vi "Table, Import from Excel Clipboard.vi"(8 "error in":errorcluster, 10 "Excel Clipboard to Import":string="TRS13058\tPower Test\t\t\t\t\nTRS13059\tAdapter Source Regulator Test \t\t\t\t\nTRS13060\t+3.3\t3.135\t3.465\tVDC\tGELE\nTRS13061\t+3.3_CONT\t3.135\t3.465\tVDC\tGELE\nTRS13062\tIVAD, ADAPTER Power Supply Current\t30\t40\tmA\tGELE\nTRS13063\tExternal Battery Source Regulator Test \t\t\t\t\nTRS13064\t+3.3\t3.135\t3.465\tVDC\tGELE\nTRS13065\t+3.3_CONT\t3.135\t3.465\tVDC\tGELE\nTRS13066\tIEXTBATT, EXT_BAT Power Supply Current\t35\t45\tmA\tGELE\nTRS13067\tInternal Battery Source Regulator Test \t\t\t\t\nTRS13068\t+3.3\t3.135\t3.465\tVDC\tGELE\nTRS13069\t+3.3_CONT\t3.135\t3.465\tVDC\tGELE\nTRS13070\tIINTBATT, INT_BAT Power Supply Current\t40\t50\tmA\tGELE\nTRS13071\t3.3V_ANALOG\t3.135\t3.465\tVDC\tGELE\nTRS13259\tReset Test\t\t\t\t\nTRS13260\tBC_RST with MR_BC_RST High\t1\t\tTTL\tEQ\nTRS13261\tBC_RST with MR_BC_RST Low\t0\t\tTTL\tEQ\nTRS13262\tMC_RST with MR_MC_RST High\t1\t\tTTL\tEQ\nTRS13263\tMC_RST with MR_MC_RST Low\t0\t\tTTL\tEQ\nTRS13072\tPower Switching\t\t\t\t\nTRS13073\tAdapter Source \t\t\t\t\nTRS13074\tVSYS\t17.1\t18.9\tVDC\tGELE\nTRS13075\tIVAD, ADAPTER Power Supply Current\t30\t40\tmA\tGELE\nTRS13076\tIEXTBATT, EXT_BAT Power Supply Current\t0\t10\tmA\tGELE\nTRS13077\tIINTBATT, INT_BAT Power Supply Current\t0\t10\tmA\tGELE\nTRS13078\tExternal Battery Source 16.8 V\t\t\t\t\nTRS13079\tVSYS\t15.96\t17.64\tVDC\tGELE\nTRS13080\tIVAD, ADAPTER Power Supply Current\t0\t10\tmA\tGELE\nTRS13081\tIEXTBATT, EXT_BAT Power Supply Current\t35\t45\tmA\tGELE\nTRS13082\tIINTBATT, INT_BAT Power Supply Current\t0\t10\tmA\tGELE\nTRS13083\tInternal Battery Source 16 V\t\t\t\t\nTRS13084\tVSYS\t15.2\t16.8\tVDC\tGELE\nTRS13085\tIVAD, ADAPTER Power Supply Current\t0\t10\tmA\tGELE\nTRS13086\tIEXTBATT, EXT_BAT Power Supply Current\t0\t10\tmA\tGELE\nTRS13087\tIINTBATT, INT_BAT Power Supply Current\t40\t50\tmA\tGELE\nTRS13109\tExternal Battery Source 16.8 V (repeat 3.3.2)\t\t\t\t\nTRS13110\tVSYS\t15.96\t17.64\tVDC\tGELE\nTRS13111\tIVAD, ADAPTER Power Supply Current\t0\t10\tmA\tGELE\nTRS13112\tIEXTBATT, EXT_BAT Power Supply Current\t25\t45\tmA\tGELE\nTRS13113\tIINTBATT, INT_BAT Power Supply Current\t0\t10\tmA\tGELE\nTRS13088\tExternal Battery Source 14.8 V\t\t\t\t\nTRS13089\tVSYS\t14.06\t15.54\tVDC\tGELE\nTRS13090\tIVAD, ADAPTER Power Supply Current\t0\t10\tmA\tGELE\nTRS13091\tIEXTBATT, EXT_BAT Power Supply Current\t40\t50\tmA\tGELE\nTRS13092\tIINTBATT, INT_BAT Power Supply Current\t0\t10\tmA\tGELE\nTRS13093\tExternal Battery Source 12.8 V\t\t\t\t\nTRS13094\tVSYS\t12.16\t13.44\tVDC\tGELE\nTRS13095\tIVAD, ADAPTER Power Supply Current\t0\t10\tmA\tGELE\nTRS13096\tIEXTBATT, EXT_BAT Power Supply Current\t45\t60\tmA\tGELE\nTRS13097\tIINTBATT, INT_BAT Power Supply Current\t0\t10\tmA\tGELE\nTRS13098\tInternal Battery Source 14 V\t\t\t\t\nTRS13099\tVSYS\t13.3\t14.7\tVDC\tGELE\nTRS13100\tIVAD, ADAPTER Power Supply Current\t0\t10\tmA\tGELE\nTRS13101\tIEXTBATT, EXT_BAT Power Supply Current\t0\t10\tmA\tGELE\nTRS13102\tIINTBATT, INT_BAT Power Supply Current\t45\t60\tmA\tGELE\nTRS13103\tInternal Battery Source 12 V\t\t\t\t\nTRS13104\tVSYS\t11.4\t12.6\tVDC\tGELE\nTRS13105\tIVAD, ADAPTER Power Supply Current\t0\t10\tmA\tGELE\nTRS13106\tIEXTBATT, EXT_BAT Power Supply Current\t0\t10\tmA\tGELE\nTRS13107\tIINTBATT, INT_BAT Power Supply Current\t50\t65\tmA\tGELE\nTRS13267\tDormant Mode Operation\t\t\t\t\nTRS13268\tInternal Battery Source 16 V\t\t\t\t\nTRS13269\tVSYS\t15.2\t16.8\tVDC\tGELE\nTRS13270\tIVAD, ADAPTER Power Supply Current\t0\t10\tmA\tGELE\nTRS13271\tIEXTBATT, EXT_BAT Power Supply Current\t0\t10\tmA\tGELE\nTRS13272\tIINTBATT, INT_BAT Power Supply Current\t40\t50\tmA\tGELE\nTRS13273\tDormant Mode\t\t\t\t\nTRS13274\tVSYS\t-0.5\t0.5\tVDC\tGELE\nTRS13275\t+3.3_CONT\t3.135\t3.465\tVDC\tGELE\nTRS13469\tExternal Power Detect\t\t\t\t\nTRS13470\tAdapter Detect\t1\t\tTTL\tEQ\nTRS13471\tEXT_BAT Detect\t1\t\tTTL\tEQ\nTRS13472\tINT_BAT Detect\t0\t\tTTL\tEQ\nTRS13108\tBooster Check\t\t\t\t\nTRS13114\tAdapter Source \t\t\t\t\nTRS13115\tVMOTOR with 0.25A Load\t17.1\t18.9\tVDC\tGELE\nTRS13264\tVMOTOR_DRIVER with 0.25A Load\t12.04\t12.54\tVDC\tGELE\nTRS13116\tVMOTOR with 0.5A Load\t17.1\t18.9\tVDC\tGELE\nTRS13265\tVMOTOR_DRIVER with 0.5A Load\t12.04\t12.54\tVDC\tGELE\nTRS13117\tVMOTOR with 1.0A Load\t17.1\t18.9\tVDC\tGELE\nTRS13266\tVMOTOR_DRIVER with 1.0A Load\t12.04\t12.54\tVDC\tGELE\nTRS13118\tExternal Battery Source 16.8 V\t\t\t\t\nTRS13119\tVMOTOR with 0.25A Load\t17.64\t18.36\tVDC\tGELE\nTRS13120\tVMOTOR with 0.5A Load\t17.64\t18.36\tVDC\tGELE\nTRS13121\tVMOTOR with 1.0A Load\t17.64\t18.36\tVDC\tGELE\nTRS13122\tInternal Battery Source 16 V\t\t\t\t\nTRS13123\tVMOTOR with 0.25A Load\t17.64\t18.36\tVDC\tGELE\nTRS13124\tVMOTOR with 0.5A Load\t17.64\t18.36\tVDC\tGELE\nTRS13125\tVMOTOR with 1.0A Load\t17.64\t18.36\tVDC\tGELE\nTRS13126\tExternal Battery Source 16.8 V\t\t\t\t\nTRS13127\tVMOTOR with 0.25A Load\t17.64\t18.36\tVDC\tGELE\nTRS13128\tVMOTOR with 0.5A Load\t17.64\t18.36\tVDC\tGELE\nTRS13129\tVMOTOR with 1.0A Load\t17.64\t18.36\tVDC\tGELE\nTRS13130\tExternal Battery Source 14.8 V\t\t\t\t\nTRS13131\tVMOTOR with 0.25A Load\t17.64\t18.36\tVDC\tGELE\nTRS13132\tVMOTOR with 0.5A Load\t17.64\t18.36\tVDC\tGELE\nTRS13133\tVMOTOR with 1.0A Load\t17.64\t18.36\tVDC\tGELE\nTRS13134\tExternal Battery Source 12.8 V\t\t\t\t\nTRS13135\tVMOTOR with 0.25A Load\t17.64\t18.36\tVDC\tGELE\nTRS13136\tVMOTOR with 0.5A Load\t17.64\t18.36\tVDC\tGELE\nTRS13137\tVMOTOR with 1.0A Load\t17.64\t18.36\tVDC\tGELE\nTRS13138\tInternal Battery Source 14 V\t\t\t\t\nTRS13139\tVMOTOR with 0.25A Load\t17.64\t18.36\tVDC\tGELE\nTRS13140\tVMOTOR with 0.5A Load\t17.64\t18.36\tVDC\tGELE\nTRS13141\tVMOTOR with 1.0A Load\t17.64\t18.36\tVDC\tGELE\nTRS13142\tInternal Battery Source 12 V\t\t\t\t\nTRS13143\tVMOTOR with 0.25A Load\t17.64\t18.36\tVDC\tGELE\nTRS13144\tVMOTOR with 0.5A Load\t17.64\t18.36\tVDC\tGELE\nTRS13145\tVMOTOR with 1.0A Load\t17.64\t18.36\tVDC\tGELE\nTRS13146\tAdapter Source (repeat step 3.6.1?)\t\t\t\t\nTRS13147\tVMOTOR with 0.25A Load\t17.64\t18.36\tVDC\tGELE\nTRS13148\tVMOTOR with 0.5A Load\t17.64\t18.36\tVDC\tGELE\nTRS13149\tVMOTOR with 1.0A Load\t17.64\t18.36\tVDC\tGELE\nTRS13633\tMotor Driver Test\t\t\t\t\nTRS13634\tStator A Phase U and Phase V\t\t\t\t\nTRS13635\tPhase U to V\t17.64\t18.36\tVDC\tGELE\nTRS13636\tPhase V to U\t-18.36\t-17.64\tVDC\tGELE\nTRS13637\tStator A Phase U and Phase W\t\t\t\t\nTRS13638\tPhase U to W\t17.64\t18.36\tVDC\tGELE\nTRS13639\tPhase W to U\t-18.36\t-17.64\tVDC\tGELE\nTRS13640\tStator A Phase V and Phase W\t\t\t\t\nTRS13641\tPhase V to W\t17.64\t18.36\tVDC\tGELE\nTRS13642\tPhase W to V\t-18.36\t-17.64\tVDC\tGELE\nTRS13634\tSTATOR B Phase U and Phase V\t\t\t\t\nTRS13635\tPhase U to V\t17.64\t18.36\tVDC\tGELE\nTRS13636\tPhase V to U\t-18.36\t-17.64\tVDC\tGELE\nTRS13637\tSTATOR B Phase U and Phase W\t\t\t\t\nTRS13638\tPhase U to W\t17.64\t18.36\tVDC\tGELE\nTRS13639\tPhase W to U\t-18.36\t-17.64\tVDC\tGELE\nTRS13640\tSTATOR B Phase V and Phase W\t\t\t\t\nTRS13641\tPhase V to W\t17.64\t18.36\tVDC\tGELE\nTRS13642\tPhase W to V\t-18.36\t-17.64\tVDC\tGELE\n", 11 "Tbl Refnum":refnum<vi>) -> (0 "error out":errorcluster, 3 "Tbl Refnumout":refnum<vi>)   [LabVIEW 2010]
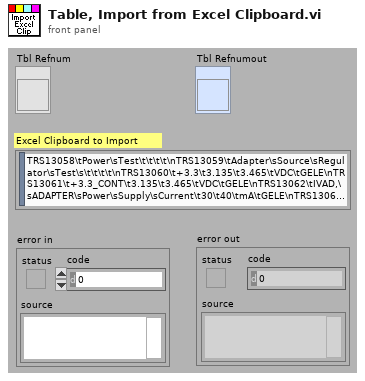
[diagram p1: front panel]
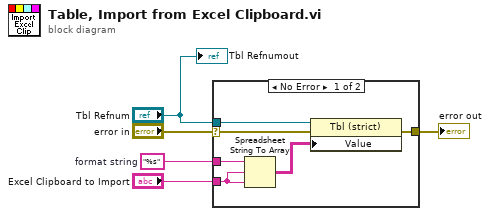
[diagram p0: block diagram]
diagram:
  w5 = "%s"  # format string
  n1 = case shown="No Error" "error in" {
    selector: "error in" -> [w6 w12]
    tunnel: w5 -> [w10 _]
    tunnel: "Excel Clipboard to Import" -> [w9 _]
    tunnel: [w8 w12] -> w3
    tunnel: "Tbl Refnum" -> [w7 _]
    frame No Error {
      n2 = Spreadsheet String To Array(format string=w10, spreadsheet string=w9, array type (2D Dbl)=w9) -> (array=w11:string[][])  [unwired: 1 in]
      n3 = property class="Tbl (strict)"(reference=w7, error in=w6, "Value"=w11) -> (error out=w8:errorcluster)  [unwired: 1 out]
    }
    frame Error {
    }
  }
  "error out" <- w3
  "Tbl Refnumout" <- "Tbl Refnum"
